vi "Lab Ventilation.vi"(1 "Paint Spraying by South West Fan":bool, 2 "Ventilation %":dbl) -> (0 "Scan Comments":string)   [LabVIEW 2022 SP3]
uses:
  Anemometry/Anemometry Sub Vis/Globals/EnFlo_Tunnel_Global.vi
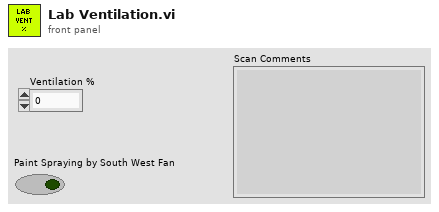
[diagram p1: front panel]
types:
  T1 = typedef "Ch_description_ADAM.ctl" = cluster{"Ch Name":string, "Type":T2, "Function":T3, "Ch State":T4, "Calibration type":T5, "A":dbl, "B":dbl, "C":dbl, "D":dbl, "Comments":string, "Address":T6, "String":string, "Duty":u16}
  T2 = typedef "Module_type_ADAM.ctl" = string
  T3 = typedef "Function_ADAM.ctl" = enum16{"Analogue Input", "Digital Input", "Event counter", "Event rate", "Analogue Output", "Digital Output", "Relay Output"}
  T4 = typedef "Channel_State.ctl" = enum16{"On", "Off", "Always On", "Always Off"}
  T5 = typedef "Calib_type_ADAM.ctl" = string
  T6 = typedef "Address.ctl" = cluster{"Main":i32, "Ch.":i32, "Sub":i32, "Port Name":string}
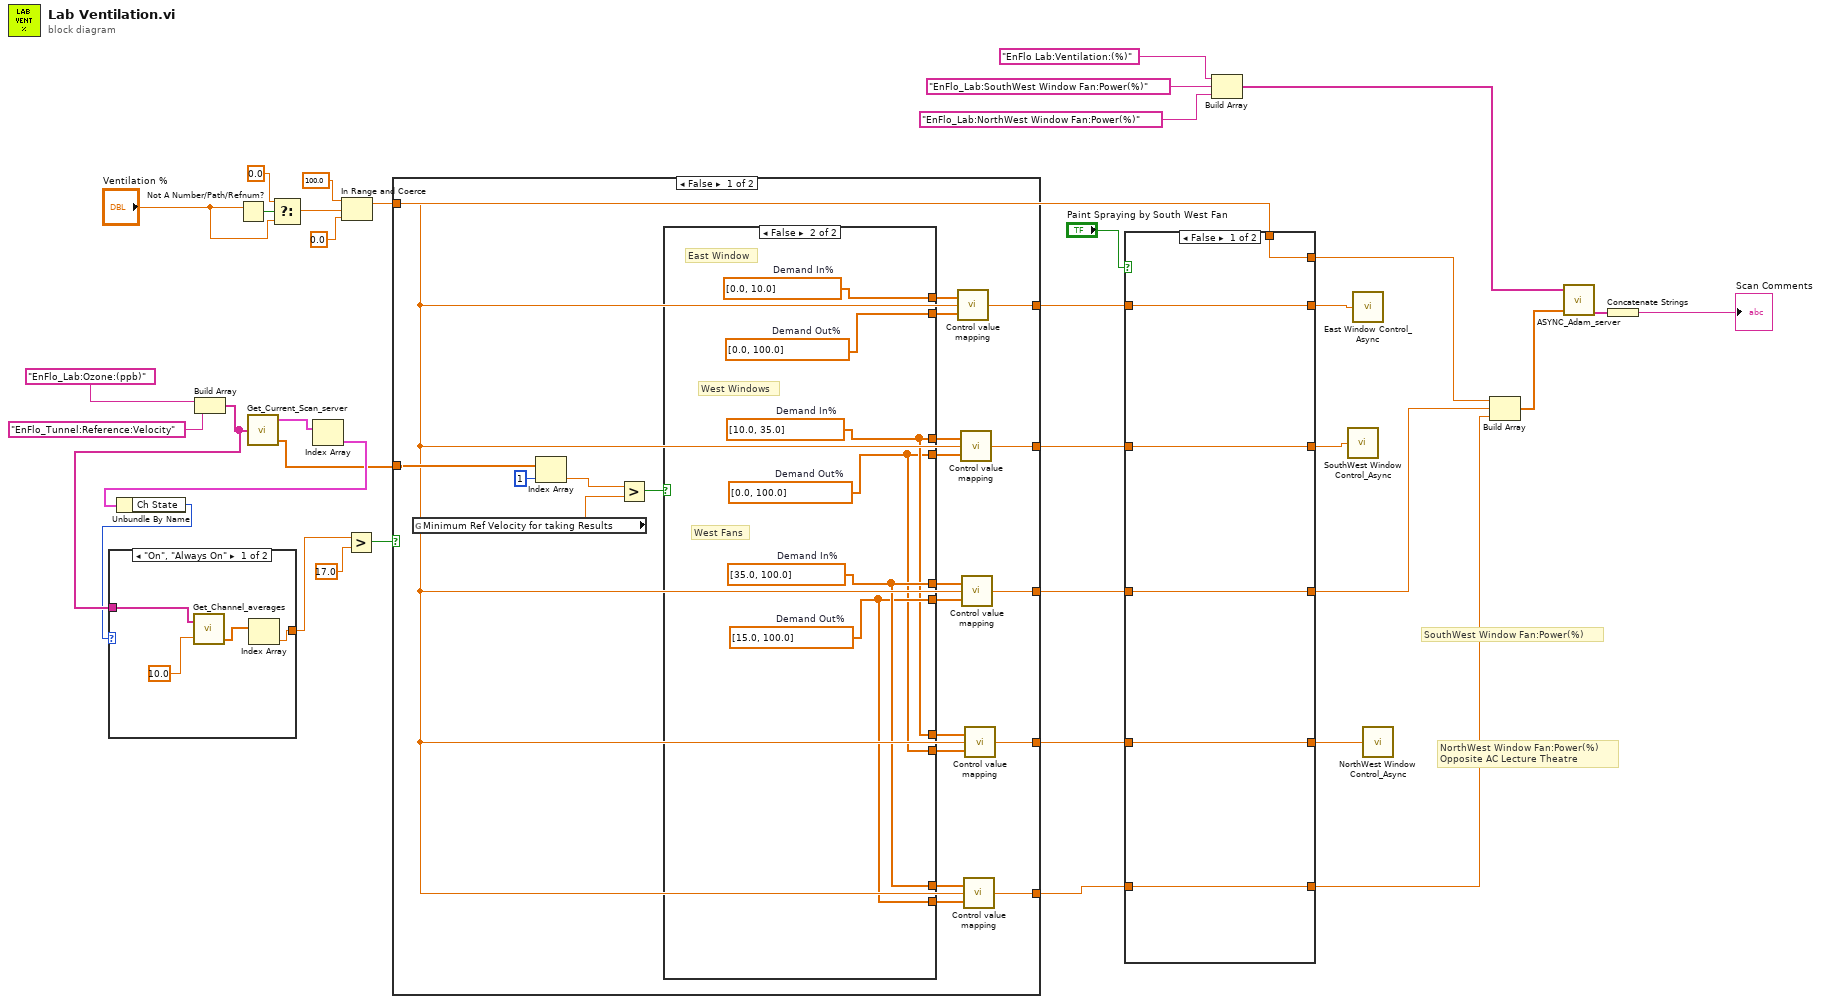
[diagram p0: block diagram]
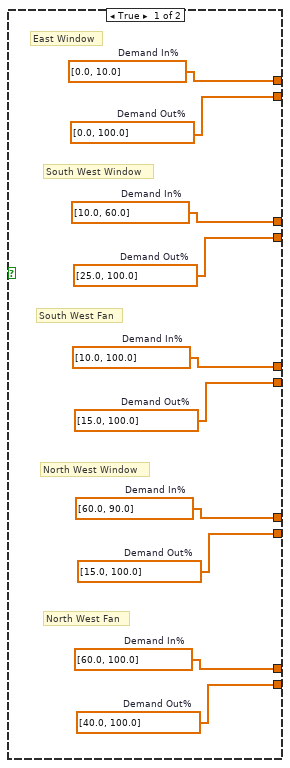
[diagram p2: hidden frame]
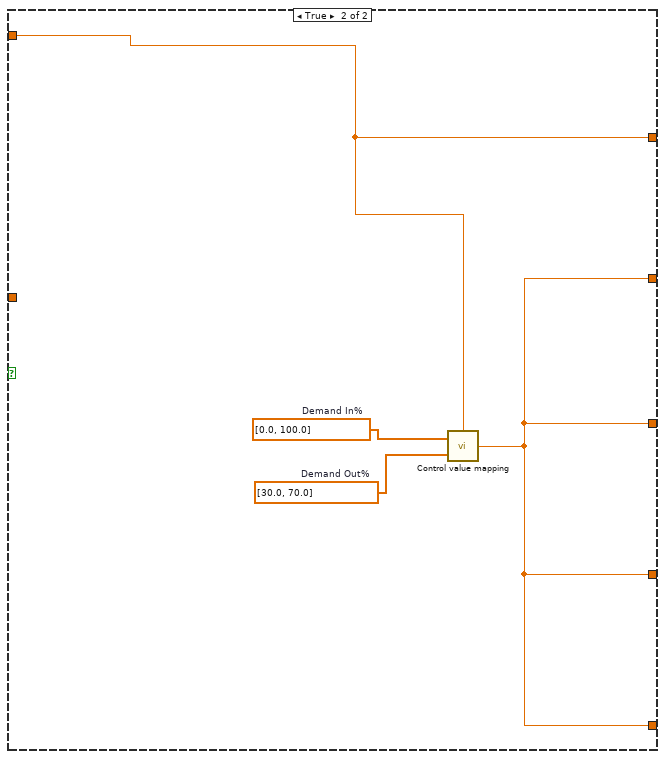
[diagram p3: hidden frame]
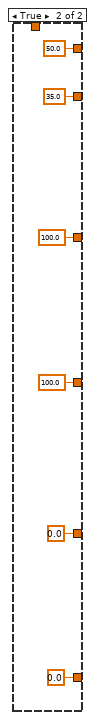
[diagram p4: hidden frame]
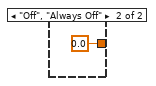
[diagram p5: hidden frame]
diagram:
  # "NorthWest Window Fan:Power(%)\nOpposite AC Lecture Theatre"
  # "SouthWest Window Fan:Power(%)"
  n1 = Build Array("EnFlo_Lab:Ozone:(ppb)", "EnFlo_Tunnel:Reference:Velocity") -> (w20:string[])
  n2 = Not A Number/Path/Refnum?(number/path/refnum="Ventilation %") -> (NaN/Path/Refnum?=w34:bool)
  n3 = call "Get_Current_Scan_server.vi"("Desired Channels"=w20) -> ("Ch Description Array"=w22:T1[], "Numerical Values"=w16:dbl[])  [unwired: 1 out]
  n4 = Select(t=0.0, s=w34, f="Ventilation %") -> (s? t:f=w30:dbl)
  n5 = Index Array(array=w22) -> (element=w21:T1)  [unwired: 1 in]
  n6 = Unbundle By Name(w21) -> ("Ch State"=w19:T4)
  n7 = case shown="\"On\", \"Always On\"" w19 {
    tunnel: w20 -> [w40 _]
    tunnel: [w38 0.0] -> w18
    frame "On", "Always On" {
      n8 = call "Get_Channel_averages.vi"("Desired Ch Names"=w40, "Averaging time (mins)"=10.0) -> ("number"=w39:dbl[])  [unwired: 1 in, 2 out]
      n9 = Index Array(array=w39) -> (element=w38:dbl)  [unwired: 1 in]
    }
    frame "Off", "Always Off" {
    }
  }
  n10 = In Range and Coerce(upper limit=100.0, x=w30, lower limit=0.0) -> (coerced(x)=w29:dbl)  [unwired: 1 out]
  n11 = Greater?(x=w18, y=17.0) -> (0:w15:bool)
  n12 = case shown="False" w15 {
    tunnel: w16 -> [w52 _]
    tunnel: [w47 w80] -> w11
    tunnel: [w46 w79] -> w9
    tunnel: [w45 w79] -> w7
    tunnel: [w44 w79] -> w5
    tunnel: [w43 w79] -> w3
    tunnel: w29 -> [w42 w80]
    frame False {
      n13 = global read "EnFlo_Tunnel_Global.vi" "Minimum Ref Velocity for taking Results"() -> (w49:dbl)
      n14 = Index Array(array=w52, index=1) -> (element=w50:dbl)
      n15 = Greater?(x=w50, y=w49) -> (0:w48:bool)
      n16 = case shown="False" w48 {
        tunnel: [w72 w78] -> w62
        tunnel: [w71 w77] -> w61
        tunnel: [w70 w74] -> w60
        tunnel: [w69 w73] -> w59
        tunnel: [w68 w75] -> w58
        tunnel: [w67 w76] -> w57
        tunnel: [w66 w74] -> w56
        tunnel: [w65 w73] -> w55
        tunnel: [w64 w75] -> w54
        tunnel: [w63 w76] -> w53
        frame True {
          w64 = dbl[] [40.0, 100.0]  # Demand Out%
          w63 = dbl[] [60.0, 100.0]  # Demand In%
          w65 = dbl[] [15.0, 100.0]  # Demand Out%
          w66 = dbl[] [60.0, 90.0]  # Demand In%
          w68 = dbl[] [15.0, 100.0]  # Demand Out%
          w67 = dbl[] [10.0, 100.0]  # Demand In%
          w69 = dbl[] [25.0, 100.0]  # Demand Out%
          w70 = dbl[] [10.0, 60.0]  # Demand In%
          w72 = dbl[] [0.0, 100.0]  # Demand Out%
          w71 = dbl[] [0.0, 10.0]  # Demand In%
          # "North West Fan"
          # "South West Fan"
          # "North West Window"
          # "South West Window"
          # "East Window"
        }
        frame False {
          w75 = dbl[] [15.0, 100.0]  # Demand Out%
          w76 = dbl[] [35.0, 100.0]  # Demand In%
          w73 = dbl[] [0.0, 100.0]  # Demand Out%
          w74 = dbl[] [10.0, 35.0]  # Demand In%
          w78 = dbl[] [0.0, 100.0]  # Demand Out%
          w77 = dbl[] [0.0, 10.0]  # Demand In%
          # "West Fans"
          # "West Windows"
          # "East Window"
        }
      }
      n17 = call "Control value mapping.vi"("Control In%"=w42, "Demand Out%"=w62, "Demand In%"=w61) -> ("Control Out%"=w47:dbl)
      n18 = call "Control value mapping.vi"("Control In%"=w42, "Demand Out%"=w59, "Demand In%"=w60) -> ("Control Out%"=w46:dbl)
      n19 = call "Control value mapping.vi"("Control In%"=w42, "Demand Out%"=w58, "Demand In%"=w57) -> ("Control Out%"=w45:dbl)
      n20 = call "Control value mapping.vi"("Control In%"=w42, "Demand Out%"=w54, "Demand In%"=w53) -> ("Control Out%"=w43:dbl)
      n21 = call "Control value mapping.vi"("Control In%"=w42, "Demand Out%"=w55, "Demand In%"=w56) -> ("Control Out%"=w44:dbl)
    }
    frame True {
      w82 = dbl[] [30.0, 70.0]  # Demand Out%
      w81 = dbl[] [0.0, 100.0]  # Demand In%
      n22 = call "Control value mapping.vi"("Control In%"=w80, "Demand Out%"=w82, "Demand In%"=w81) -> ("Control Out%"=w79:dbl)
    }
  }
  n23 = case shown="False" "Paint Spraying by South West Fan" {
    tunnel: [w88 35.0 ("Control Out%")] -> w12
    tunnel: w11 -> [w88 _]
    tunnel: [w87 100.0 ("Control Out%")] -> w10
    tunnel: w9 -> [w87 _]
    tunnel: [w86 100.0 ("Control Out%")] -> w8
    tunnel: w7 -> [w86 _]
    tunnel: [w85 0.0 ("Control Out%")] -> w6
    tunnel: w5 -> [w85 _]
    tunnel: [w84 0.0 ("Control Out%")] -> w4
    tunnel: w3 -> [w84 _]
    tunnel: [w83 50.0 ("upper limit")] -> w2
    tunnel: w29 -> [w83 _]
    frame False {
    }
    frame True {
    }
  }
  n24 = Build Array("EnFlo Lab:Ventilation:(%)", "EnFlo_Lab:SouthWest Window Fan:Power(%)", "EnFlo_Lab:NorthWest Window Fan:Power(%)") -> (w27:string[])
  n25 = call "SouthWest Window Control_Async.vi"("Desired Window Open %"=w10) -> ()  [unwired: 1 in]
  n26 = call "East Window Control_Async.vi"("Desired Window Open %"=w12) -> ()  [unwired: 1 in]
  n27 = call "NorthWest Window Control_Async.vi"("Desired Window Open %"=w6) -> ()  [unwired: 1 in]
  n28 = Build Array(w2, w8, w4) -> (w14:dbl[])
  n29 = call "ASYNC_Adam_server.vi"("Values"=w14, "Channel Names"=w27) -> ("Scan Comments"=w13:string[])  [unwired: 1 in, 2 out]
  n30 = Concatenate Strings(w13) -> (→"Scan Comments":string)
